vi "Start.vi"   [LabVIEW 2014]
uses:
  Application/SmartPalette/Palette.vi
  Application/SmartPalette/SmartPalette.lvlib
types:
  T1 = enum32{"Invalid", "Standard", "Closed", "Hidden", "Minimized", "Maximized"}
  T2 = enum32{"Bad", "Idle", "Run top level", "Running"}
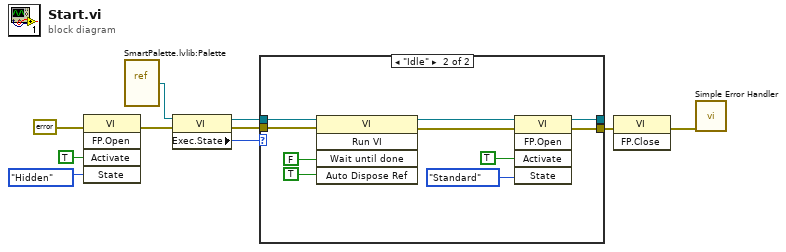
[diagram p0: block diagram]
diagram:
  n1 = invoke class="VI" method="FP.Open"(error in=errorcluster {"status"=FALSE, "code"=0, "source"=""} ("error in (no error)"), "Activate"=TRUE, "State"=T1."Hidden") -> (error out=w3:errorcluster)  [unwired: 2 in, 4 out]
  n2 = vi-ref "SmartPalette.lvlib:Palette.vi"() -> (w10:refnum<vi>)
  n3 = property class="VI"(reference=w10, error in=w3) -> (reference out=w7:refnum<vi>, error out=w8:errorcluster, "Exec.State"=w9:T2)
  n4 = case shown="\"Idle\"" w9 {
    tunnel: w8 -> [w11 w22]
    tunnel: w7 -> [w12 w21]
    tunnel: [w12 w15] -> _
    tunnel: [w11 w17] -> w6
    frame Default {
    }
    frame "Idle" {
      n5 = invoke class="VI" method="Run VI"(reference=w21, error in=w22, "Wait until done"=FALSE, "Auto Dispose Ref"=TRUE) -> (reference out=w16:refnum<vi>, error out=w18:errorcluster)  [unwired: 1 in, 3 out]
      n6 = invoke class="VI" method="FP.Open"(reference=w16, error in=w18, "Activate"=TRUE, "State"=T1."Standard") -> (reference out=w15:refnum<vi>, error out=w17:errorcluster)  [unwired: 1 in, 3 out]
    }
  }
  n7 = invoke class="VI" method="FP.Close"(error in=w6) -> (error out=w5:errorcluster)  [unwired: 2 in, 2 out]
  n8 = call <vilib>:"Simple Error Handler.vi"("error in (no error)"=w5) -> ()  [unwired: 4 in, 5 out]
